vi "H5D Write 1D Integer.vi"(8 "error in (no error)":errorcluster, 9 "close?":bool, 10 "new data":u64[](array[numeric]), 11 "dataset_id":i32) -> (0 "error out":errorcluster, 3 "dup dataset_id":i32)   [LabVIEW 2011]
doc: "This VI adds new data to the end of an existing vector. It is useful for streaming data to disk. It is also used to close datasets, when called with <B>close?</B> equal TRUE and an empty input dataset."
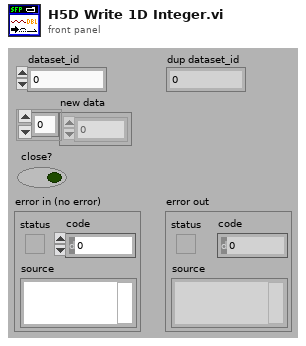
[diagram p1: front panel]
types:
  T1 = typedef "DU64 2U32.ctl" = cluster{"high bytes":u32, "low bytes":u32}
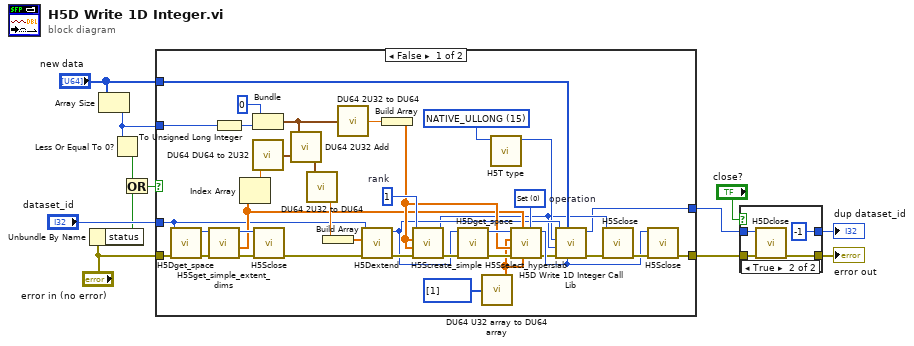
[diagram p0: block diagram]
diagram:
  n1 = Unbundle By Name("error in (no error)") -> ("status"=w1:bool)
  n2 = Array Size(array="new data") -> (size(s)=w5:i32)
  n3 = Less Or Equal To 0?(x=w5) -> (x <= 0?=w2:bool)
  n4 = Or(x=w2, y=w1) -> (x .or. y?=w3:bool)
  n5 = case shown="False" w3 {
    tunnel: "error in (no error)" -> [w50 w52]
    tunnel: w5 -> [w47 _]
    tunnel: "new data" -> [w20 _]
    tunnel: "dataset_id" -> [w24 w51]
    tunnel: [w15 w51] -> w9
    tunnel: [w22 w52] -> w6
    frame False {
      w21 = 15 items=["None", "IEEE_F32BE", "IEEE_F32LE", "IEEE_F64BE", "IEEE_F64LE", "NATIVE_CHAR", "NATIVE_SCHAR", "NATIVE_UCHAR", "NATIVE_SHORT", "NATIVE_USHORT", "NATIVE_INT", "NATIVE_UINT", "NATIVE_LONG", "NATIVE_ULONG", "NATIVE_LLONG", "NATIVE_ULLONG", "NATIVE_FLOAT", "NATIVE_DOUBLE", "NATIVE_LDOUBLE", "NATIVE_B8", "NATIVE_B16", "NATIVE_B32", "NATIVE_B64", "NATIVE_OPAQUE", "NATIVE_HADDR", "NATIVE_HSIZE", "NATIVE_HSSIZE", "NATIVE_HERR", "NATIVE_HBOOL", "STD_U8LE", "STD_U8BE", "STD_U16LE", "STD_U16BE", "STD_U32LE", "STD_U32BE", "STD_U64LE", "STD_U64BE", "STD_B8LE", "STD_B8BE", "STD_B16LE", "STD_B16BE", "STD_B32LE", "STD_B32BE", "STD_B64LE", "STD_B64BE", "STD_REF_OBJ", "STD_REF_DSETREG", "C_S1", "STD_I8LE", "STD_I8BE", "STD_I16LE", "STD_I16BE", "STD_I32LE", "STD_I32BE", "STD_I64LE", "STD_I64BE", ""] ("defined type")
      w32 = 0 items=["Set", "OR"]  # operation
      w37 = 1  # rank
      n6 = call <instrlib>:"H5Dget_space.vi"("error in (no error)"=w50, "dataset_id"=w24) -> ("error out"=w49:errorcluster, "space_id"=w48:i32)  [unwired: 8 in]
      n7 = call <instrlib>:"H5Sget_simple_extent_dims.vi"("error in (no error)"=w49, "space_id"=w48) -> ("error out"=w43:errorcluster, "DU64 dims"=w27:dbl[], "dup space_id"=w42:i32)  [unwired: 5 in, 2 out]
      n8 = To Unsigned Long Integer(number=w47) -> (unsigned 32bit integer=w46:u32)
      n9 = Index Array(array=w27) -> (element=w30:dbl)  [unwired: 1 in]
      n10 = Bundle("Cluster Element"=u32 0, w46) -> (w26:cluster{"Cluster Element":u32, u32})  [unwired: 1 in]
      n11 = call <instrlib>:"DU64 DU64 to 2U32.vi"("DU64"=w30) -> ("2U32"=w25:T1)
      n12 = call <instrlib>:"H5Sclose.vi"("error in (no error)"=w43, "space_id"=w42) -> ("error out"=w40:errorcluster)  [unwired: 9 in]
      n13 = call <instrlib>:"DU64 2U32 Add.vi"("Input 2"=w25, "Input 1"=w26) -> ("sum"=w44:T1)
      n14 = call <instrlib>:"DU64 2U32 to DU64.vi"("2U32"=w44) -> ("DU64"=w41:dbl)
      n15 = Build Array(w41) -> (w39:dbl[])
      n16 = call <instrlib>:"DU64 2U32 to DU64.vi"("2U32"=w26) -> ("DU64"=w36:dbl)
      n17 = call <instrlib>:"H5Dextend.vi"("error in (no error)"=w40, "DU64 size"=w39, "dataset_id"=w24) -> ("error out"=w38:errorcluster, "dup dataset_id"=w19:i32)  [unwired: 7 in]
      n18 = Build Array(w36) -> (w31:dbl[])
      n19 = call <instrlib>:"H5Screate_simple.vi"("error in (no error)"=w38, "DU64 maxdims"=w31, "DU64 dims"=w31, "rank"=w37) -> ("error out"=w35:errorcluster, "space_id"=w17:i32)  [unwired: 6 in]
      n20 = call <instrlib>:"H5Dget_space.vi"("error in (no error)"=w35, "dataset_id"=w19) -> ("error out"=w34:errorcluster, "space_id"=w33:i32)  [unwired: 8 in]
      n21 = call <instrlib>:"DU64 U32 array to DU64 array.vi"("U32 array"=u32[] [1]) -> ("DU64 array"=w28:dbl[])
      n22 = call <instrlib>:"H5T type.vi"("defined type"=w21) -> ("type_id"=w18:i32)  [unwired: 10 in]
      n23 = call <instrlib>:"H5Sselect_hyperslab.vi"("operation"=w32, "DU64 block"=w28, "DU64 start"=w27, "error in (no error)"=w34, "DU64 count"=w31, "DU64 stride"=w28, "space_id"=w33) -> ("error out"=w13:errorcluster, "dup space_id"=w16:i32)  [unwired: 3 in]
      n24 = call "H5D Write 1D Integer Call Lib.vi"("file_space_id"=w16, "buf"=w20, "error in (no error)"=w13, "mem_space_id"=w17, "mem_type_id"=w18, "dataset_id"=w19) -> ("error out"=w14:errorcluster, "dup dataset_id"=w15:i32)  [unwired: 4 in]
      n25 = call <instrlib>:"H5Sclose.vi"("error in (no error)"=w14, "space_id"=w17) -> ("error out"=w23:errorcluster)  [unwired: 9 in]
      n26 = call <instrlib>:"H5Sclose.vi"("error in (no error)"=w23, "space_id"=w16) -> ("error out"=w22:errorcluster)  [unwired: 9 in]
    }
    frame True {
    }
  }
  n27 = case shown="True" "close?" {
    tunnel: [w53 w58] -> w10
    tunnel: w9 -> [w54 w57]
    tunnel: [w54 -1 ("dup dataset_id")] -> w7
    tunnel: w6 -> [w53 w55]
    frame False {
    }
    frame True {
      n28 = call <instrlib>:"H5Dclose.vi"("error in (no error)"=w55, "dataset_id"=w57) -> ("error out"=w58:errorcluster)  [unwired: 9 in]
    }
  }
  "dup dataset_id" <- w7
  "error out" <- w10
